vi "CameraLoop.vi"(8 "error in":errorcluster, 9 "Image In":T1, 10 "Settings (Clamp (Rake))":T3={"Contrast"=16, "Filter width"=10, "Steepness"=63, "Subsampling Ratio"=30, "Show Search Area"=TRUE, "Show Search Lines"=TRUE, "Show Edges Found"=TRUE, "Show Result"=TRUE}, 11 "Inputs":T4={"File Name"="", "Force (Hz)"=0.0, "Camera (Hz)"=0.0, "Systole (V)"=0.0, "Diastole (V)"=0.0, "T (sec)"=0.0, "Delay (sec)"=0.0, "Setpoint Function"=enum."Incremental PWM Step", "Max Diam (mm)"=0.0, "DAQmx Servo Task"="MyPulseOutputTask", "Force Sensor Channel"="Dev2/ai7", "DAQmx LED Task"="MyDigitalOutTask", "Camera Selector"="cam5", "FS Task Out"="", "Servo Task Out"="", "LED Task Out"="", "Camera Session Out"="", "Color Pane"=0} {"Color Pane" items=["Blue", "Red", "Green", "Saturation", "Value", "Intensity", "Luminance", "Hue", ""]}) -> (0 "error out":errorcluster, 1 "Image Out":T1, 2 "Diameter Cluster":T2, 3 "Image Dst Out":T1, 5 "Diameter Exceeded?":bool)   [LabVIEW 2020]
uses:
  Controls/Inputs.ctl
  Controls/Serpoint.ctl
  <vilib>/userDefined/High Color/IMAQdx.ctl
  <vilib>/vision/Image Controls.llb/IMAQ Image.ctl
  <vilib>/vision/driver/NI_Vision_Acquisition_Software.lvlib
  <vilib>/vision/NI_Vision_Development_Module.lvlib
panel:
  # "Test Variables:"
  # "Sampling Frequencies:"
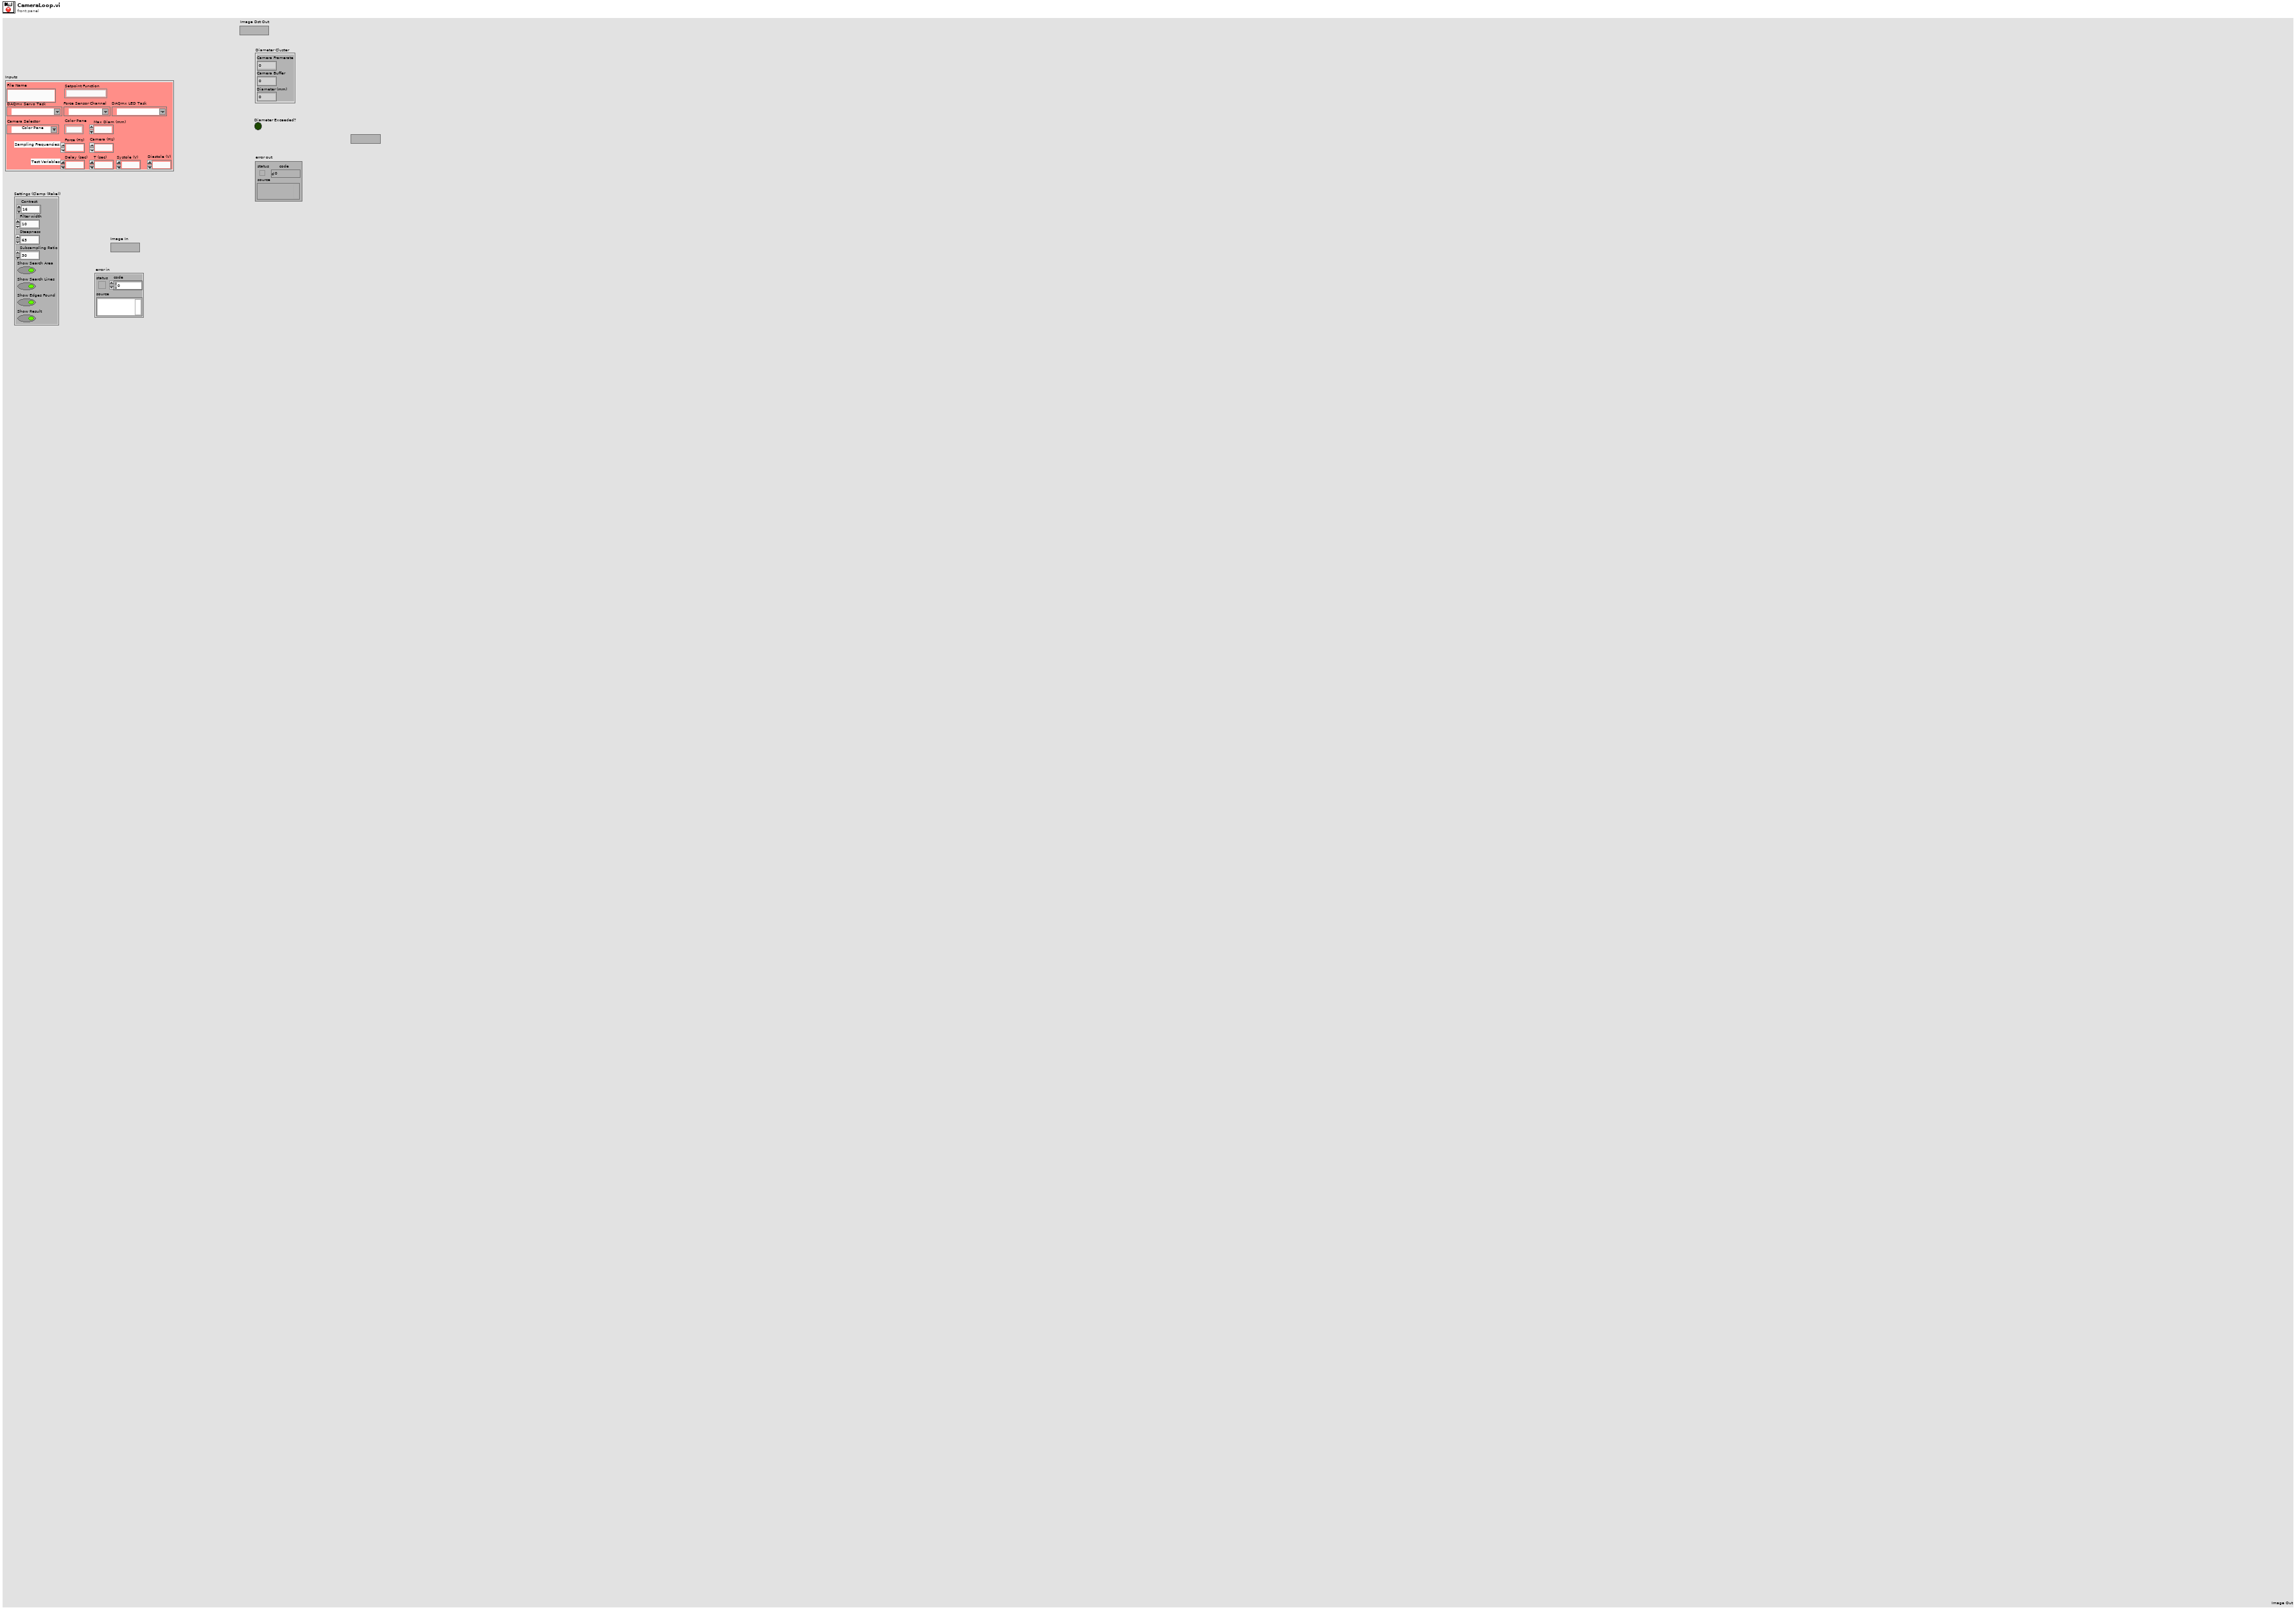
[diagram p1: front panel]
types:
  T1 = typedef "IMAQ Image.ctl" = refnum<image>
  T2 = cluster{"Camera Framerate":dbl, "Camera Buffer":u32, "Diameter (mm)":dbl}
  T3 = cluster{"Contrast":i32, "Filter width":i32, "Steepness":i32, "Subsampling Ratio":u32, "Show Search Area":bool, "Show Search Lines":bool, "Show Edges Found":bool, "Show Result":bool}
  T4 = typedef "Inputs.ctl" = cluster{"File Name":string, "Force (Hz)":dbl, "Camera (Hz)":dbl, "Systole (V)":dbl, "Diastole (V)":dbl, "T (sec)":dbl, "Delay (sec)":dbl, "Setpoint Function":T5, "Max Diam (mm)":dbl, "DAQmx Servo Task":refnum<k21>, "Force Sensor Channel":tag, "DAQmx LED Task":refnum<k21>, "Camera Selector":T6, "FS Task Out":refnum<k21>, "Servo Task Out":refnum<k21>, "LED Task Out":refnum<k21>, "Camera Session Out":T6, "Color Pane":i32}
  T5 = typedef "Serpoint.ctl" = enum16{"Incremental PWM Step", "PWM Step", "Ramp", "Sinusoidal", "Blood-Pressure"}
  T6 = typedef "IMAQdx.ctl" = refnum<k21>
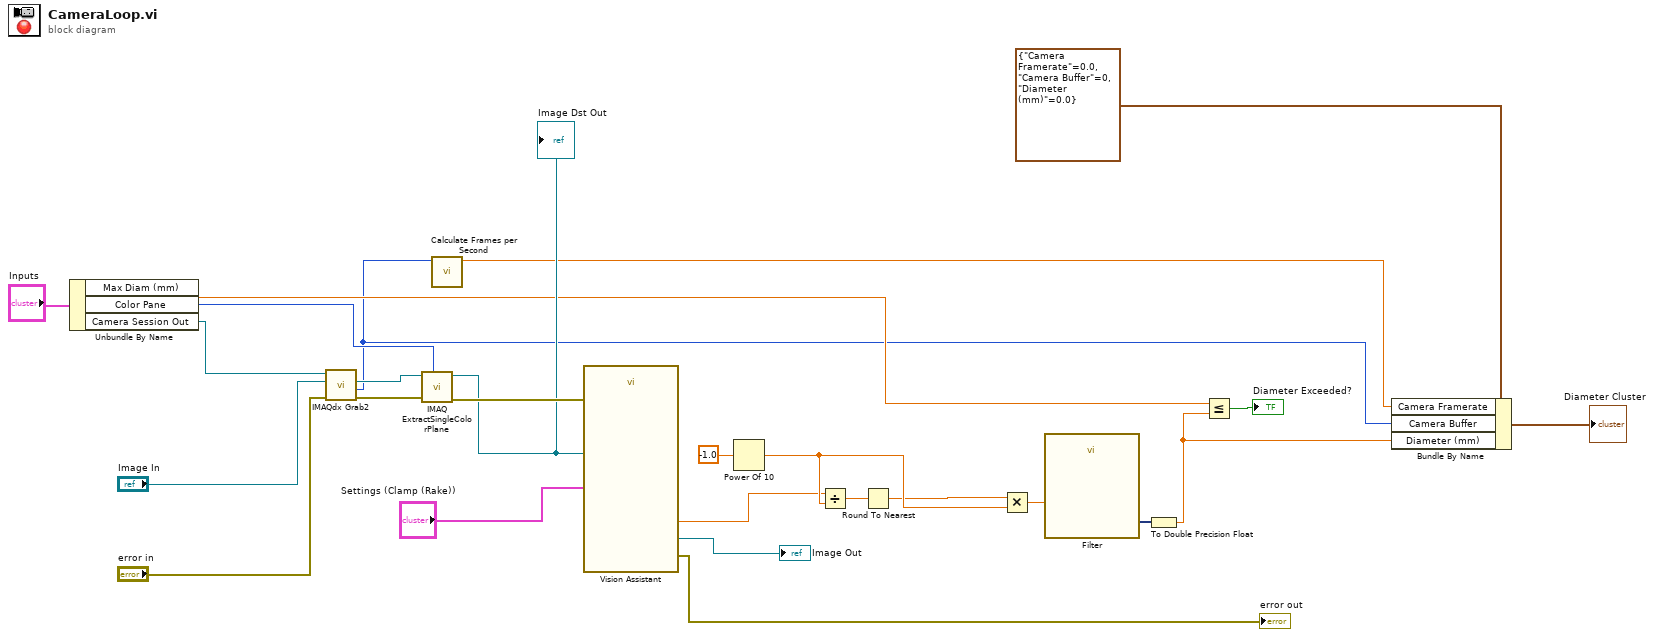
[diagram p0: block diagram]
diagram:
  n1 = Unbundle By Name("Inputs") -> ("Max Diam (mm)"=w10:dbl, "Color Pane"=w21:i32, "Camera Session Out"=w2:T6)
  n2 = call <vilib>:"IMAQdx Grab2.vi"("error in"="error in", "Image In"="Image In", "Session In"=w2) -> ("error out"=w25:errorcluster, "Buffer Number Out"=w5:u32, "Image Out"=w22:T1)  [unwired: 5 in, 1 out]
  n3 = call "IMAQ ExtractSingleColorPlane"("Color Plane"=w21, "error in (no error)"=w25, "Image Src"=w22) -> ("error out"=w26:errorcluster, "Image Dst Out"=w23:T1)  [unwired: 7 in]
  "Image Dst Out" <- w23
  n4 = call <vilib>:"Calculate Frames per Second.vi"("Buffer Number"=w5) -> ("Acquired Frames/s"=w6:dbl)  [unwired: 8 in, 2 out]
  n5 = call "Vision Assistant"("Image In"=w23, "Settings (Clamp (Rake) 1)"="Settings (Clamp (Rake))", "error in"=w26) -> ("Image Out"=→"Image Out":T1, "Distance (calibrated) (Clamp (Rake) 1)"=w12:sgl, "error out"=→"error out":errorcluster)  [unwired: 21 in, 1 out]
  n6 = Power Of 10(x=-1.0 ("Power of ten")) -> (10^x=w15:dbl)
  n7 = Divide(x=w12, y=w15) -> (x/y=w13:dbl)
  n8 = Round To Nearest(number=w13) -> (nearest integer value=w14:dbl)
  n9 = Multiply(x=w14, y=w15) -> (x*y=w17:dbl)
  n10 = call "Filter"("Signal"=w17) -> ("Filtered Signal"=w11:dynamicdata)  [unwired: 9 in, 1 out]
  n11 = To Double Precision Float(number=w11) -> (double precision float=w4:dbl)
  n12 = Less Or Equal? ("Does diameter exceed max diam?")(x=w10, y=w4) -> (x <= y?=→"Diameter Exceeded?":bool)
  n13 = Bundle By Name(cluster=T2 {"Camera Framerate"=0.0, "Camera Buffer"=0, "Diameter (mm)"=0.0} ("input cluster"), "Camera Framerate"=w6, "Camera Buffer"=w5, "Diameter (mm)"=w4) -> (→"Diameter Cluster":T2)
